vi "configureA.vi"(5 "Reset":bool, 6 "Order":T1(array[cluster]), 7 "Path Properties":T4(array[cluster]), 8 "Rectangle Properties":T5(array[cluster]), 9 "Funnel Propeties":T2(array[cluster]), 10 "Inkscape File Path":path) -> (0 "Image Size":cluster{"Width":dbl, "Height":dbl}, 1 "boolean array":bool[](array[boolean]), 2 "string array":string[](array[string]), 3 "shape properties":T3(array[cluster]), 4 "boolean":bool)   [LabVIEW 2013]
uses:
  Global Variables.vi
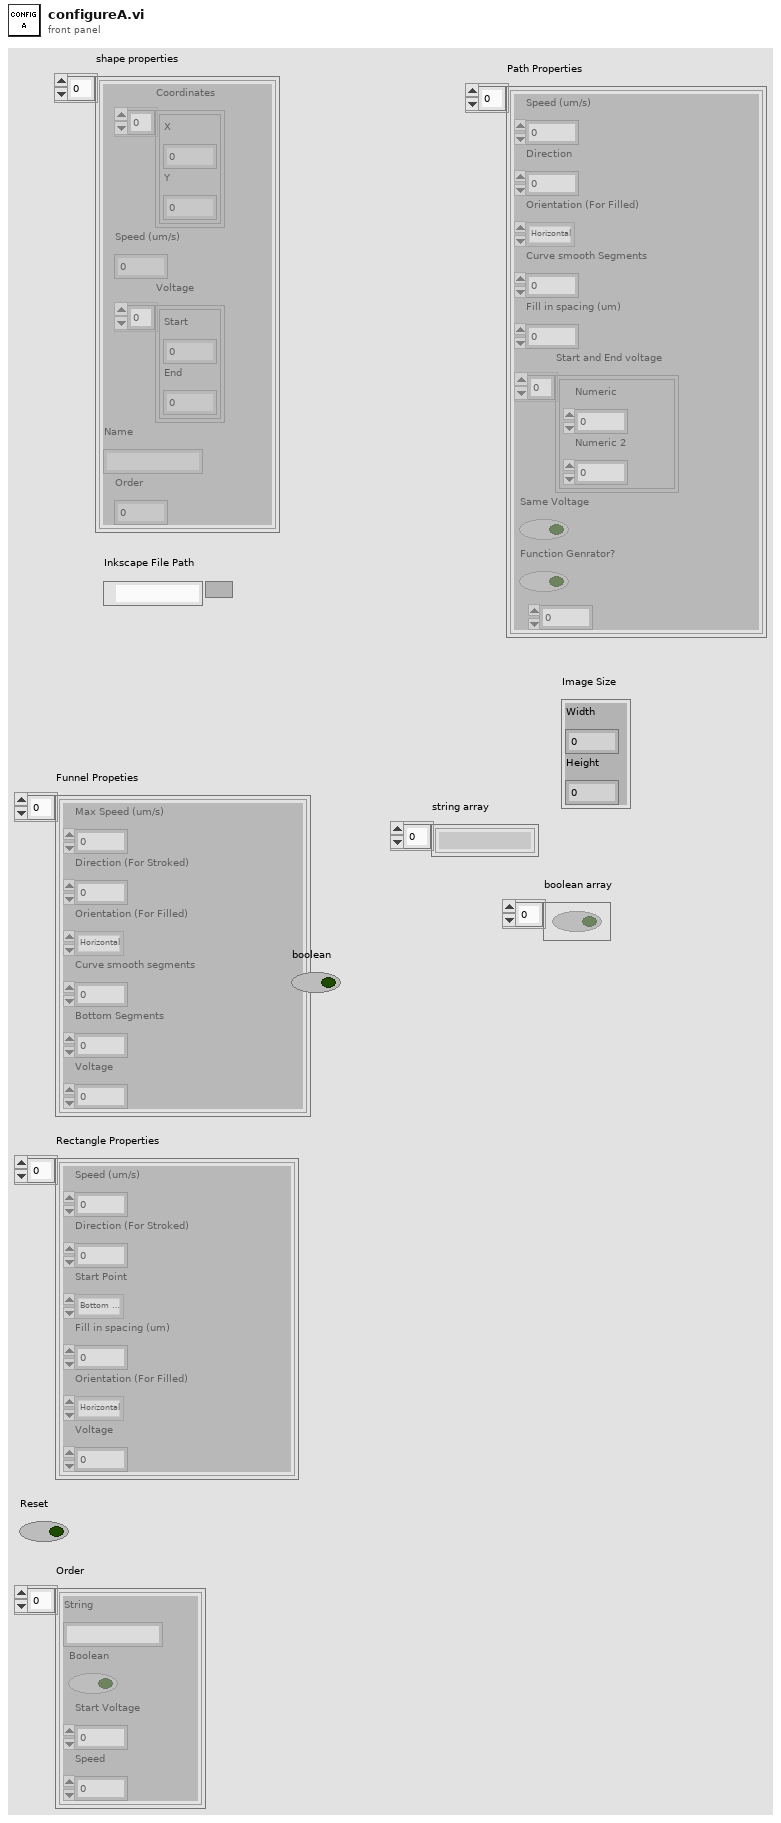
[diagram p1: front panel]
types:
  T1 = cluster{"String":string, "Boolean":bool, "Start Voltage":dbl, "Speed":dbl}[]
  T2 = cluster{"Max Speed (um/s)":dbl, "Direction (For Stroked)":u16, "Orientation (For Filled)":enum16{"Horizontal", "Vertical"}, "Curve smooth segments":dbl, "Bottom Segments":dbl, "Voltage":dbl}[]
  T3 = cluster{"Coordinates":cluster{"X":dbl, "Y":dbl}[], "Speed (um/s)":dbl, "Voltage":cluster{"Start":dbl, "End":dbl}[], "Name":string, "Order":i32}[]
  T4 = cluster{"Speed (um/s)":dbl, "Direction":u16, "Orientation (For Filled)":enum16{"Horizontal", "Vertical"}, "Curve smooth Segments":dbl, "Fill in spacing (um)":dbl, "Start and End voltage":cluster{"Numeric":dbl, "Numeric 2":dbl}[], "Same Voltage":bool, "Function Genrator?":bool, "Function generator #":dbl}[]
  T5 = cluster{"Speed (um/s)":dbl, "Direction (For Stroked)":u16, "Start Point":enum16{"Bottom Left Corner", "Bottom Right Corner", "Top Left Corner", "Top Right Corner"}, "Fill in spacing (um)":dbl, "Orientation (For Filled)":enum16{"Horizontal", "Vertical"}, "Voltage":dbl}[]
  T6 = typedef "NI_Matrix.lvlib/RealMatrix.ctl" = dbl[][]
  T7 = cluster{"Fill Color":string, "Stroke Color":string, "Width":dbl, "Height":dbl, "X":dbl, "Y":dbl, "Transformation Matrix":T6}[]
  T8 = cluster{"XML":string, "XML":string, "Array of Commands":cluster{"Command Type":string, "Coordinates":cluster{"X":dbl, "Y":dbl}[]}[], "Transformation Matrix":T6, "Order":i32}[]
  T9 = cluster{cluster{"X":dbl, "Y":dbl}[], "Max Speed (um/s)":dbl, "Voltage":cluster{"Voltage":dbl, "Voltage":dbl}[], "Name":string, "Order":i32}[]
  T10 = cluster{cluster{"X":dbl, "Y":dbl}[], "Speed (um/s)":dbl, "Voltage":cluster{"Start":dbl, "End":dbl}[], "Name":string, "Order":i32}[]
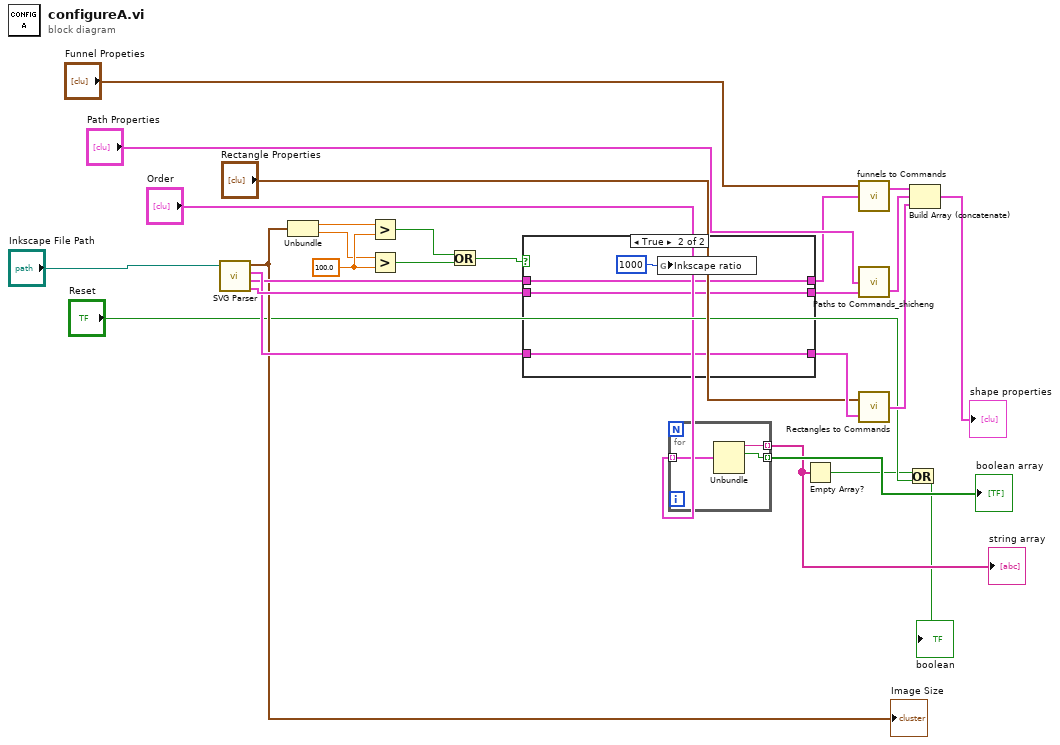
[diagram p0: block diagram]
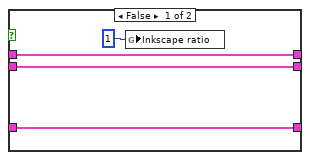
[diagram p2: hidden frame]
diagram:
  w14 = 100.0 ("y")
  n1 = call "SVG Parser.vi"("XML File Path"="Inkscape File Path") -> ("Image Size"=w11:cluster{"Width":dbl, "Height":dbl}, "rects"=w19:T7, "Funnel"=w18:T8, "Path"=w24:T8)  [unwired: 2 in, 1 out]
  "Image Size" <- w11
  n2 = Unbundle(w11) -> ("Width"=w12:dbl, "Height"=w13:dbl)
  n3 = Greater?(x=w12, y=w14) -> (0:w15:bool)
  n4 = Greater?(x=w13, y=w14) -> (0:w16:bool)
  n5 = Or(x=w15, y=w16) -> (x .or. y?=w17:bool)
  n6 = case shown="True" w17 {
    tunnel: w19 -> [w29 w35]
    tunnel: w18 -> [w31 w34]
    tunnel: w24 -> [w30 w33]
    tunnel: [w29 w35] -> w27
    tunnel: [w31 w34] -> w20
    tunnel: [w30 w33] -> w21
    frame False {
      n7 = global write "Global Variables.vi" "Inkscape ratio"(1) -> ()
    }
    frame True {
      n8 = global write "Global Variables.vi" "Inkscape ratio"(1000) -> ()
    }
  }
  n9 = for {
    tunnel: "Order" -> [w38] mode=indexing
    tunnel: [w37] -> w5 mode=indexing
    tunnel: [w36] -> w6 mode=indexing
    n10 = Unbundle(w38) -> ("String"=w37:string, "Boolean"=w36:bool)  [unwired: 2 out]
  }
  "boolean array" <- w6
  "string array" <- w5
  n11 = Empty Array?(array=w5) -> (empty?=w3:bool)
  n12 = call "funnels to Commands.vi"("Funnel"=w20, "Funnel Propeties"="Funnel Propeties") -> ("Lithography information"=w8:T9)  [unwired: 2 in]
  n13 = call "Paths to Commands_shicheng.vi"("Path"=w21, "Path Properties"="Path Properties") -> ("Lithography information"=w9:T10)  [unwired: 1 in, 1 out]
  n14 = call "Rectangles to Commands.vi"("rects"=w27, "Rectangle Properties"="Rectangle Properties") -> ("Lithography information"=w26:T3)
  n15 = Or(x=w3, y="Reset") -> (x .or. y?=→"boolean":bool)
  n16 = Build Array (concatenate)(w8, w9, w26) -> (→"shape properties":T3)
